vi "SET MAG for Blue.vi"(8 "error in (no error)":errorcluster, 11 "stack name":string="DB/Button 1") -> (0 "error out":errorcluster, 3 "Heading":dbl)   [LabVIEW 2023]
uses:
  <vilib>/Rock Robotics/Network Tables/NT Read Boolean.vi
  Global INIT.vi
  Global odometry.vi
  <vilib>/Rock Robotics/Network Tables/NT Write String.vi
  <vilib>/Rock Robotics/Network Tables/NT Write Boolean.vi
panel:
  out "IMU OFFSET (deg)":dbl=-90.0
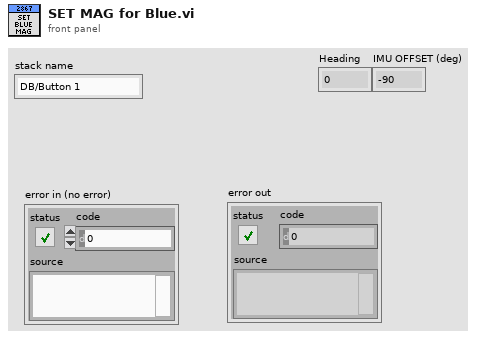
[diagram p1: front panel]
types:
  T1 = cluster{"Yaw":dbl, "Roll":dbl, "Pitch":dbl, "Heading":dbl, "Fused Heading":dbl}
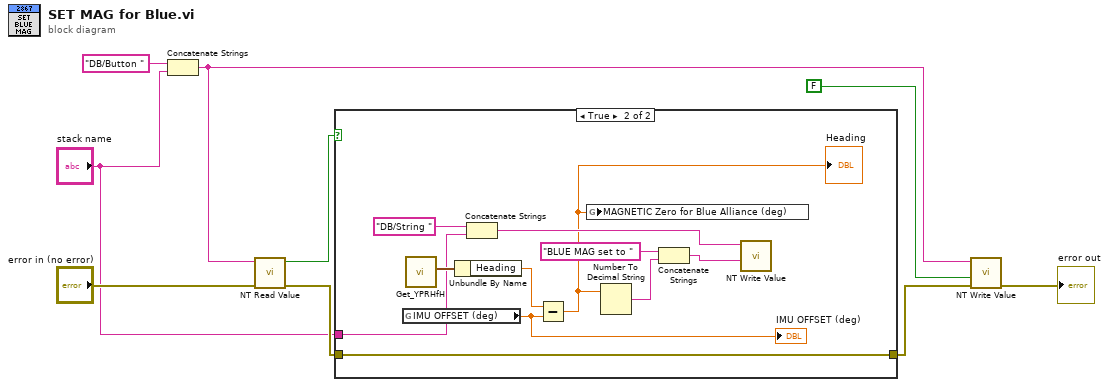
[diagram p0: block diagram]
diagram:
  n1 = Concatenate Strings("DB/Button " ("string"), "stack name") -> (w2:string)
  n2 = call-poly <vilib>:"NT Read Value.vi"("error in"="error in (no error)", "name"=w2) -> ("error out"=w5:errorcluster, "value"=w9:bool)  [unwired: 7 in, 1 out]
  n3 = case shown="True" w9 {
    tunnel: w5 -> [_ w20]
    tunnel: [_ w20] -> w4
    tunnel: "stack name" -> [_ w14]
    frame False {
    }
    frame True {
      n4 = global read "Global INIT.vi" "IMU OFFSET (deg)"() -> (w10:dbl)
      "IMU OFFSET (deg)" <- w10
      n5 = call <vilib>:"Get_YPRHfH.vi"() -> ("YRPHfH"=w19:T1)  [unwired: 11 in]
      n6 = Unbundle By Name(w19) -> ("Heading"=w12:dbl)
      n7 = Concatenate Strings("DB/String " ("string"), w14) -> (w17:string)
      n8 = Subtract(x=w12, y=w10) -> (x-y=w11:dbl)
      "Heading" <- w11
      n9 = global write "Global odometry.vi" "MAGNETIC Zero for Blue Alliance (deg)"(w11) -> ()
      n10 = Number To Decimal String(number=w11) -> (decimal integer string=w13:string)  [unwired: 1 in]
      n11 = Concatenate Strings("BLUE MAG set to " ("string"), w13) -> (w15:string)
      n12 = call-poly <vilib>:"NT Write Value.vi"("value"=w15, "name"=w17) -> ()  [unwired: 9 in, 1 out]
    }
  }
  n13 = call-poly <vilib>:"NT Write Value.vi"("error in"=w4, "value"=FALSE, "name"=w2) -> ("error out"=→"error out":errorcluster)  [unwired: 8 in]
